vi "LidarData.vi"(11 "LIDAR IN":refnum<visa-resource-name>) -> (0 "LIDAR Data":cluster{"Magnitude":dbl[], "Direction":dbl[]}, 3 "LIDAR Out":refnum<visa-resource-name>)   [LabVIEW 2011]
doc: "This example shows how to configure the URG to aquire data and then creates a polar graph using the magnitude and direction arrays.\n\nTo use this example with a USB LIDAR on a cRIO target, change the VISA resource name type to USB Raw. See the help for the control for additional information."
uses:
  <instrlib>/Hokuyo URG Series/Hokuyo URG Series.lvlib
panel:
  in  "Encoding Width":u16(ring)=3 items=["2 Byte"=2, "3 Byte"=3]
  in  "Cluster Count":dbl=1.0
  in  "Start Point":dbl=-120.0
  in  "End Point":dbl=120.0
  in  "polar attributes (hidden)":T1={"maximum"=30000.0, "minimum"=0.0, "clip to min"=FALSE, "log?(F)"=TRUE, "grid color"=6710886, "plot color"=65280, "fmt and prec"={"format"=enum."Decimal", "precision"=0}, "visible section"=8} {"minimum" format="%0.2f"; "maximum" format="%0.2f"}
  # "Measurement Configuration"
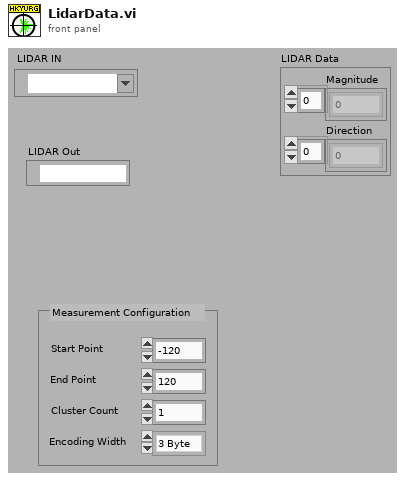
[diagram p1: front panel]
types:
  T1 = cluster{"maximum":dbl, "minimum":dbl, "clip to min":bool, "log?(F)":bool, "grid color":u32, "plot color":u32, "fmt and prec":cluster{"format":enum8{"Decimal", "Scientific", "Engineering", "Binary", "Octal", "Hex"}, "precision":u8}, "visible section":u16}
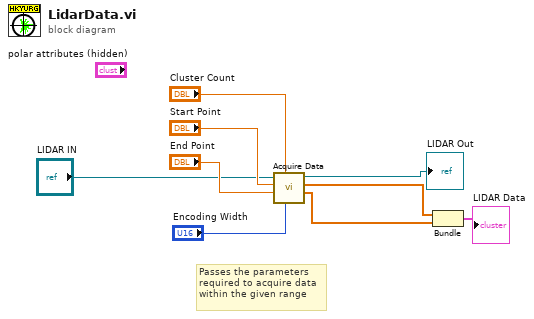
[diagram p0: block diagram]
diagram:
  # "Passes the parameters\nrequired to acquire data\nwithin the given range"
  n1 = call <instrlib>:"Acquire Data.vi"("Data Encoding Width (3 Byte)"="Encoding Width", "Cluster Count (1)"="Cluster Count", "End Point (120°)"="End Point", "Start Point (-120°)"="Start Point", "VISA resource name"="LIDAR IN") -> ("Direction"=w2:dbl[], "Magnitude"=w3:dbl[], "VISA resource name out"=→"LIDAR Out":refnum<visa-resource-name>)  [unwired: 3 in, 1 out]
  n2 = Bundle("Magnitude"=w3, "Direction"=w2) -> (→"LIDAR Data":cluster{"Magnitude":dbl[], "Direction":dbl[]})  [unwired: 1 in]
